vi "Speed 0800.vi"(10 "Speed":i32=100) -> (2 "Command":string)   [LabVIEW 2017]
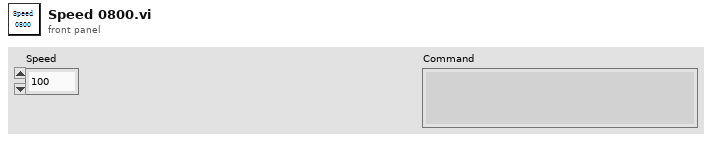
[diagram p1: front panel]
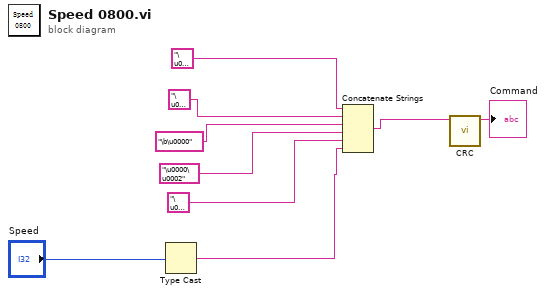
[diagram p0: block diagram]
diagram:
  n1 = Type Cast(x="Speed") -> (*(type *) &x=w3:string)  [unwired: 1 in]
  n2 = Concatenate Strings("\u0001", "\u0010", "\b\u0000", "\u0000\u0002", "\u0004", w3) -> (w2:string)
  n3 = call "CRC.vi"("字符串"=w2) -> ("连接的字符串"=→"Command":string)  [unwired: 9 in, 1 out]
